vi "Test Convert.vi"(11 "Error in":errorcluster) -> (15 "Error out":errorcluster)   [LabVIEW 2020, in "CaseConvert.lvlib"]
doc: "This VI is used for validating uppercase to lowercase and lowercase to uppercase."
uses:
  CaseConvert.lvlib
  053bf008-8162-4b8b-9ea9-ccb3880044f0.vi
  28369dab-26a1-4c6c-bd5d-27e1c6642fa2.vi
  <vilib>/addons/_JKI Toolkits/Caraya/classes/Test Suite/Define Test Suite (JUnit Report).vi
  <vilib>/SLL Drona/APIs/Stimulus/KeyBoardSimulation/KeyboardSimulationCore.vi
  <vilib>/SLL Drona/APIs/Stimulus/ControlValue/SetValueAuto.vi
  <vilib>/SLL Drona/APIs/Stimulus/KeyBoardSimulation/KeyBoardSimulationForTargetVI.vi
  <vilib>/SLL Drona/APIs/Assert/AssertControlValue/Equal.vi
  <vilib>/SLL Drona/APIs/Stimulus/VI/CloseVI.vi
  <vilib>/SLL Drona/APIs/Assert/AssertVI/AssertVIExecIdle.vi
  <vilib>/addons/_JKI Toolkits/Caraya/classes/Assert/Assert Equal Value_Variant.vi
  <vilib>/Utility/error.llb/Error Cluster From Error Code.vi
  <vilib>/ErrorRing/Error Ring.xnode
  <vilib>/addons/_JKI Toolkits/Caraya/classes/Test Suite/Test Suite.lvclass
  <vilib>/addons/_JKI Toolkits/Caraya/classes/Test/Test.lvclass
  <vilib>/SLL Drona/Drona.lvlib
  user32.dll
  <vilib>/Wiresmith Technology/G CLI/CLI Class/CLI.lvclass
  <vilib>/SLL Drona/APIs/Stimulus/KeyBoardSimulation/KeyboardSimulation.lvlib
  <vilib>/SLL Drona/APIs/Assert/AssertControlValue/AssertControlValue.lvlib
  <vilib>/SLL Drona/APIs/Stimulus/VI/VI.lvlib
  <vilib>/SLL Drona/APIs/Stimulus/ControlValue/ControlValue.lvlib
  <vilib>/SLL Drona/APIs/Assert/AssertVI/AssertVI.lvlib
  <vilib>/addons/_JKI Toolkits/Caraya/classes/Assert/Assert.lvclass
panel:
  # "CASE CONVERT TEST"
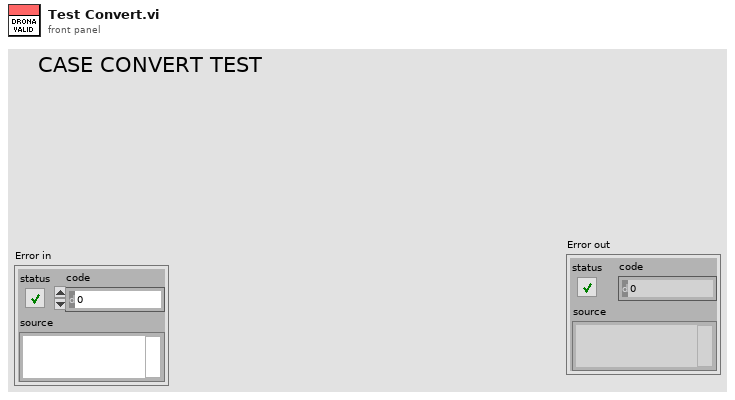
[diagram p1: front panel]
types:
  T1 = cluster{" Key":u8, "Action":enum16{"Press", "Up", "Down"}, "Delay (ms)":u32}[]
  T2 = enum32{"Invalid", "Standard", "Closed", "Hidden", "Minimized", "Maximized"}
  T3 = cluster{"Key Array":cluster{" Key":u8, "Action":enum16{"Press", "Up", "Down"}, "Delay (ms)":u32}[], "Input":string, "Output":string}[]
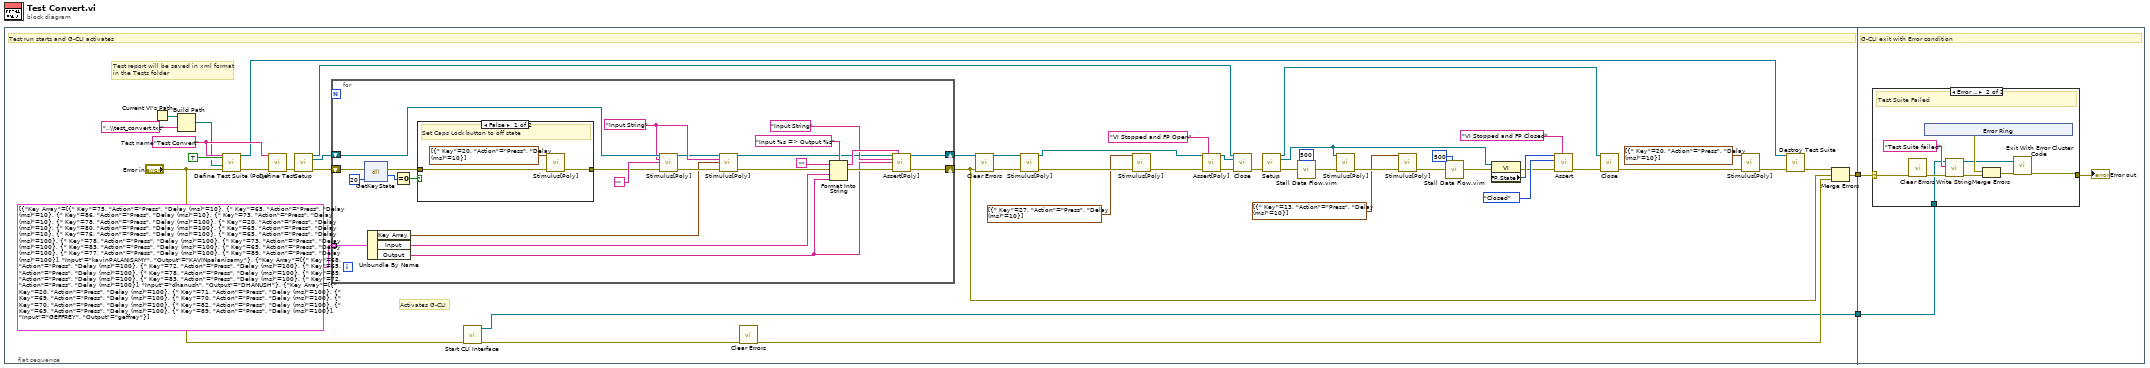
[diagram p0: block diagram]
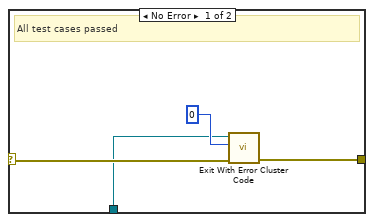
[diagram p3: hidden frame]
diagram:
  n1 = flat-sequence {
    tunnel: [w34] -> w2
    tunnel: [w31] -> w1
    tunnel: w2 -> [w79]
    tunnel: w1 -> [w80]
    frame #0 {
      w43 = "Test Convert"  # Test name
      # "Activates G-CLI"
      # "Test report will be saved in xml format\nin the Tests folder"
      # "Test run starts and G-CLI activates"
      n2 = Current VI's Path() -> (path=w41:path)
      n3 = Build Path(base path=w41, name or relative path="..\\test_convert.txt") -> (appended path=w39:path)
      n4 = call-poly <vilib>:"Define Test Suite (Poly).vi"("error in (no error)"="Error in", "Report Path"=w39, "Interactive"=TRUE, "Label (VI Title)"=w43) -> ("error out"=w44:errorcluster, "Test Suite"=w32:refnum<class "Test Suite.lvclass">)  [unwired: 5 in, 1 out]
      n5 = call <vilib>:"Define Test.vi"("error in (no error)"=w44, "Label (VI Title)"=w43) -> ("error out"=w49:errorcluster)  [unwired: 8 in, 1 out]
      n6 = call <vilib>:"Setup.vi"("error in"=w49) -> ("Application Ref"=w27:refnum<vi>, "VI Reference Out"=w46:refnum<vi>, "error out"=w47:errorcluster)  [unwired: 12 in]
      n7 = for {
        shift-right: [w66] -> w37
        shift-left: w47 -> [w55]
        shift-right: [w65] -> w48
        shift-left: w46 -> [w64]
        tunnel: T3 [{"Key Array"=[{" Key"=75, "Action"=enum."Press", "Delay (ms)"=10}, {" Key"=65, "Action"=enum."Press", "Delay (ms)"=10}, {" Key"=86, "Action"=enum."Press", "Delay (ms)"=10}, {" Key"=73, "Action"=enum."Press", "Delay (ms)"=10}, {" Key"=78, "Action"=enum."Press", "Delay (ms)"=100}, {" Key"=20, "Action"=enum."Press", "Delay (ms)"=10}, {" Key"=80, "Action"=enum."Press", "Delay (ms)"=100}, {" Key"=65, "Action"=enum."Press", "Delay (ms)"=10}, {" Key"=76, "Action"=enum."Press", "Delay (ms)"=100}, {" Key"=65, "Action"=enum."Press", "Delay (ms)"=100}, {" Key"=78, "Action"=enum."Press", "Delay (ms)"=100}, {" Key"=73, "Action"=enum."Press", "Delay (ms)"=100}, {" Key"=83, "Action"=enum."Press", "Delay (ms)"=100}, {" Key"=65, "Action"=enum."Press", "Delay (ms)"=100}, {" Key"=77, "Action"=enum."Press", "Delay (ms)"=100}, {" Key"=89, "Action"=enum."Press", "Delay (ms)"=100}], "Input"="kavinPALANISAMY", "Output"="KAVINpalanisamy"}, {"Key Array"=[{" Key"=68, "Action"=enum."Press", "Delay (ms)"=100}, {" Key"=72, "Action"=enum."Press", "Delay (ms)"=100}, {" Key"=65, "Action"=enum."Press", "Delay (ms)"=100}, {" Key"=78, "Action"=enum."Press", "Delay (ms)"=100}, {" Key"=85, "Action"=enum."Press", "Delay (ms)"=100}, {" Key"=83, "Action"=enum."Press", "Delay (ms)"=100}, {" Key"=72, "Action"=enum."Press", "Delay (ms)"=100}], "Input"="dhanush", "Output"="DHANUSH"}, {"Key Array"=[{" Key"=20, "Action"=enum."Press", "Delay (ms)"=100}, {" Key"=71, "Action"=enum."Press", "Delay (ms)"=100}, {" Key"=69, "Action"=enum."Press", "Delay (ms)"=100}, {" Key"=70, "Action"=enum."Press", "Delay (ms)"=100}, {" Key"=70, "Action"=enum."Press", "Delay (ms)"=100}, {" Key"=82, "Action"=enum."Press", "Delay (ms)"=100}, {" Key"=69, "Action"=enum."Press", "Delay (ms)"=100}, {" Key"=89, "Action"=enum."Press", "Delay (ms)"=100}], "Input"="GEFFREY", "Output"="geffrey"}] -> [w53] mode=indexing
        w63 = "Input String"
        n8 = dll-call lib="user32.dll" fn="GetKeyState"(error in=w55, "arg1"=20) -> (error out=w57:errorcluster, "return type"=w58:i32)  [unwired: 3 in, 1 out]
        n9 = Unbundle By Name(w53) -> ("Key Array"=w52:T1, "Input"=w51:string, "Output"=w50:string)
        n10 = Equal To 0?(x=w58) -> (x = 0?=w59:bool)
        n11 = case shown="False" w59 {
          tunnel: w57 -> [w76 w77]
          tunnel: [w75 w77] -> w54
          frame False {
            # "Set Caps Lock button to off state"
            n12 = call-poly <vilib>:"Stimulus[Poly].vi"("Key Array"=T1 [{" Key"=20, "Action"=enum."Press", "Delay (ms)"=10}], "error in"=w76) -> ("error out"=w75:errorcluster)  [unwired: 13 in]
          }
          frame True {
          }
        }
        n13 = call-poly <vilib>:"Stimulus[Poly].vi"("VI Reference In"=w64, "Control Path"=w63, "Value (Signaling)"="", "error in"=w54) -> ("VI Reference Out"=w60:refnum<vi>, "error out"=w61:errorcluster)  [unwired: 10 in]
        n14 = call-poly <vilib>:"Stimulus[Poly].vi"("VI Reference In"=w60, "Control Path"=w63, "Key Array"=w52, "error In"=w61) -> ("VI Reference Out"=w67:refnum<vi>, "error IO"=w68:errorcluster)  [unwired: 10 in]
        n15 = Format Into String(format string="Input %s => Output %s", initial string="", error in=w68, w51, w50) -> (resulting string=w70:string, error out=w71:errorcluster)
        n16 = call-poly <vilib>:"Assert[Poly].vi"("VI Reference In"=w67, "Test Label"=w70, "Control Path"="Input String", "Control Value"=w50, "Error In"=w71) -> ("VI Reference Out"=w65:refnum<vi>, "Error Out"=w66:errorcluster)  [unwired: 9 in]
      }
      n17 = call <vilib>:"Start CLI Interface.vi"("error in (no error)"="Error in") -> ("error out"=w36:errorcluster, "CLI out"=w34:refnum<class "CLI.lvclass">)  [unwired: 7 in, 2 out]
      n18 = call <vilib>:"Clear Errors.vi"("error in (no error)"=w36) -> ("error out"=w35:errorcluster)  [unwired: 5 in, 1 out]
      n19 = call <vilib>:"Clear Errors.vi"("error in (no error)"=w37) -> ("error out"=w45:errorcluster)  [unwired: 5 in, 1 out]
      n20 = call-poly <vilib>:"Stimulus[Poly].vi"("VI Reference In"=w48, "error in"=w45) -> ("VI Reference Out"=w24:refnum<vi>, "error out"=w30:errorcluster)  [unwired: 12 in]
      n21 = call-poly <vilib>:"Stimulus[Poly].vi"("Key Array"=T1 [{" Key"=27, "Action"=enum."Press", "Delay (ms)"=10}], "error in"=w30) -> ("error out"=w22:errorcluster)  [unwired: 13 in]
      n22 = call-poly <vilib>:"Assert[Poly].vi"("VI Reference In"=w24, "Test Label"="VI Stopped and FP Open", "Error In"=w22) -> ("VI Reference Out"=w23:refnum<vi>, "Error Out"=w21:errorcluster)  [unwired: 11 in]
      n23 = call <vilib>:"Close.vi"("Application Ref"=w27, "VI Reference"=w23, "error in"=w21) -> ("error out"=w28:errorcluster)  [unwired: 12 in]
      n24 = call <vilib>:"Setup.vi"("error in"=w28) -> ("Application Ref"=w10:refnum<vi>, "VI Reference Out"=w16:refnum<vi>, "error out"=w26:errorcluster)  [unwired: 12 in]
      n25 = call "Stall Data Flow.vim"("value in"=w26, "milliseconds to wait"=u32 500) -> ("value out"=w19:errorcluster)  [unwired: 1 out]
      n26 = call-poly <vilib>:"Stimulus[Poly].vi"("VI Reference In"=w16, "error in"=w19) -> ("error out"=w18:errorcluster)  [unwired: 12 in, 1 out]
      n27 = call-poly <vilib>:"Stimulus[Poly].vi"("Key Array"=T1 [{" Key"=13, "Action"=enum."Press", "Delay (ms)"=10}], "error in"=w18) -> ("error out"=w15:errorcluster)  [unwired: 13 in]
      n28 = call "Stall Data Flow.vim"("value in"=w15, "milliseconds to wait"=u32 500) -> ("value out"=w8:errorcluster)  [unwired: 1 out]
      n29 = property class="VI"(reference=w16, error in=w8) -> (error out=w12:errorcluster, "FP.State"=w14:T2)  [unwired: 1 out]
      n30 = call-poly <vilib>:"Assert.vi"("Label"="VI Stopped and FP Closed", "error in (no error)"=w12, "Y"=T2."Closed" ("Front Panel Window:State"), "X"=w14) -> ("error out"=w11:errorcluster)  [unwired: 6 in, 1 out]
      n31 = call <vilib>:"Close.vi"("Application Ref"=w10, "error in"=w11) -> ("error out"=w4:errorcluster)  [unwired: 13 in]
      n32 = call-poly <vilib>:"Stimulus[Poly].vi"("Key Array"=T1 [{" Key"=20, "Action"=enum."Press", "Delay (ms)"=10}], "error in"=w4) -> ("error out"=w3:errorcluster)  [unwired: 13 in]
      n33 = call-dynamic "Destroy Test Suite.vi"("error in (no error)"=w3, "Test Suite in"=w32) -> ("error out"=w33:errorcluster)  [unwired: 8 in, 1 out]
      n34 = Merge Errors(w33, w37, w35) -> (w31:errorcluster)
    }
    frame #1 {
      # "G-CLI exit with Error condition"
      n35 = case shown="Error .." w80 {
        selector: w80 -> [w84 w91]
        tunnel: [w82 w93] -> w78
        tunnel: w79 -> [w81 w85]
        frame No Error {
          # "All test cases passed"
          n36 = call <vilib>:"Exit With Error Cluster Code.vi"("error in (no error)"=w84, "No Error Code (0)"=0, "CLI in"=w81) -> ("error out"=w82:errorcluster)  [unwired: 8 in]
        }
        frame Error {
          # "Test Suite Failed"
          n37 = call <vilib>:"Clear Errors.vi"("error in (no error)"=w91) -> ("error out"=w90:errorcluster)  [unwired: 5 in, 1 out]
          n38 = xnode "Error Ring"() -> ("error out"=w89:errorcluster)
          n39 = call <vilib>:"Write String.vi"("error in (no error)"=w90, "Text to Write"="Test Suite failed", "CLI in"=w85) -> ("error out"=w88:errorcluster, "CLI out"=w86:refnum<class "CLI.lvclass">)  [unwired: 7 in]
          n40 = Merge Errors(w89, w88) -> (w87:errorcluster)
          n41 = call <vilib>:"Exit With Error Cluster Code.vi"("error in (no error)"=w87, "CLI in"=w86) -> ("error out"=w93:errorcluster)  [unwired: 9 in]
        }
      }
      "Error out" <- w78
    }
  }
